vi "Shift Point by Samples.vi"(5 "Buffer Length":i32, 7 "dt":dbl, 8 "error in (no error)":errorcluster, 10 "Samples":i32, 11 "Data Point in":T1) -> (0 "error out":errorcluster, 2 "Samples dup":i32, 3 "Data Point out":T1)   [LabVIEW 2015, in "Waveform Data Logger Engine.lvlib" / "Waveform Buffer.lvclass"]
uses:
  Waveform Buffer.lvclass
  Data Point.ctl
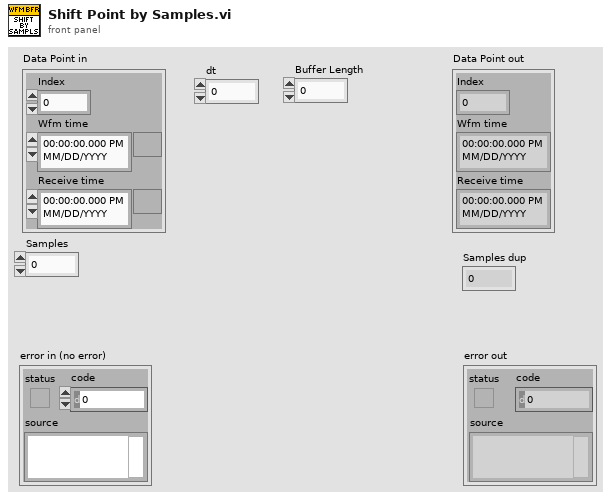
[diagram p1: front panel]
types:
  T1 = typedef "Waveform Data Logger Engine.lvlib/Waveform Buffer.lvclass/Data Point.ctl" = cluster{"Index":i32, "Wfm time":timestamp, "Receive time":timestamp}
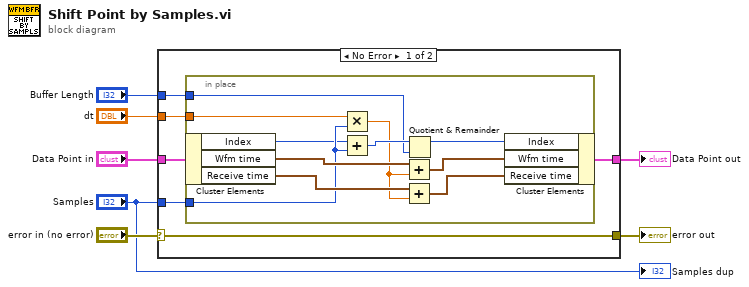
[diagram p0: block diagram]
diagram:
  n1 = case shown="No Error" "error in (no error)" {
    selector: "error in (no error)" -> [w13 w26]
    tunnel: [w13 w26] -> w6
    tunnel: [w8 w25] -> w4
    tunnel: "Data Point in" -> [w12 w25]
    tunnel: "dt" -> [w11 _]
    tunnel: "Buffer Length" -> [w10 _]
    tunnel: "Samples" -> [w9 _]
    frame No Error {
      n2 = in-place {
        in-place-border: w9 -> [w16]
        in-place-border: w11 -> [w22]
        in-place-border: w10 -> [w14]
        n3 = in-place-cluster #1(w12) -> ("Index"=w15:i32, "Wfm time"=w21:timestamp, "Receive time"=w20:timestamp)
        n4 = Multiply(x=w22, y=w16) -> (x*y=w17:dbl)
        n5 = Add(x=w15, y=w16) -> (x+y=w24:i32)
        n6 = Add(x=w21, y=w17) -> (x+y=w18:timestamp)
        n7 = Add(x=w20, y=w17) -> (x+y=w19:timestamp)
        n8 = Quotient & Remainder(x=w24, y=w14) -> (x-y*floor(x/y)=w23:i32)  [unwired: 1 out]
        n9 = in-place-cluster #1("Index"=w23, "Wfm time"=w18, "Receive time"=w19) -> (w8:T1)
      }
    }
    frame Error {
    }
  }
  "error out" <- w6
  "Data Point out" <- w4
  "Samples dup" <- "Samples"
